vi "Circular.vi"(5 "Direction":u16(ring) items=["Clockwise", "Counter-clockwise"], 7 "Speed":dbl, 8 "error in (no error)":errorcluster, 9 "XY End":dbl[](array[numeric]), 10 "XY Center":dbl[](array[numeric]), 11 "Gantry in":refnum<class "A3200.lvclass">) -> (0 "error out":errorcluster, 3 "Gantry out":refnum<class "A3200.lvclass">)   [LabVIEW 2016, in "A3200.lvclass"]
uses:
  A3200.lvclass
  A3200.lvclass/A3200.ctl
  <userlib>/Aerotech A3200.lnk/Aerotech VIs.lvlib
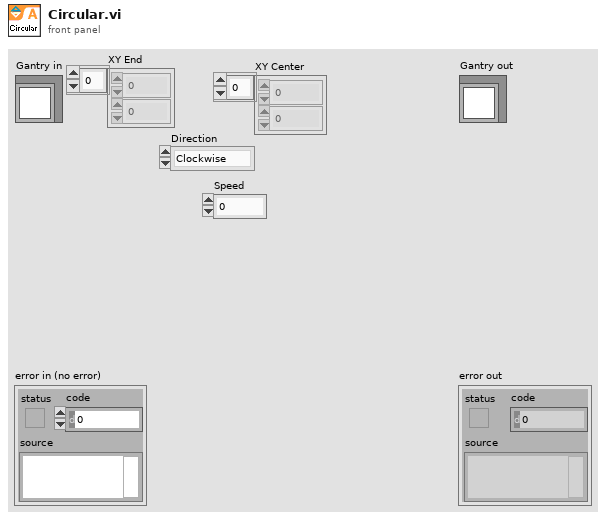
[diagram p1: front panel]
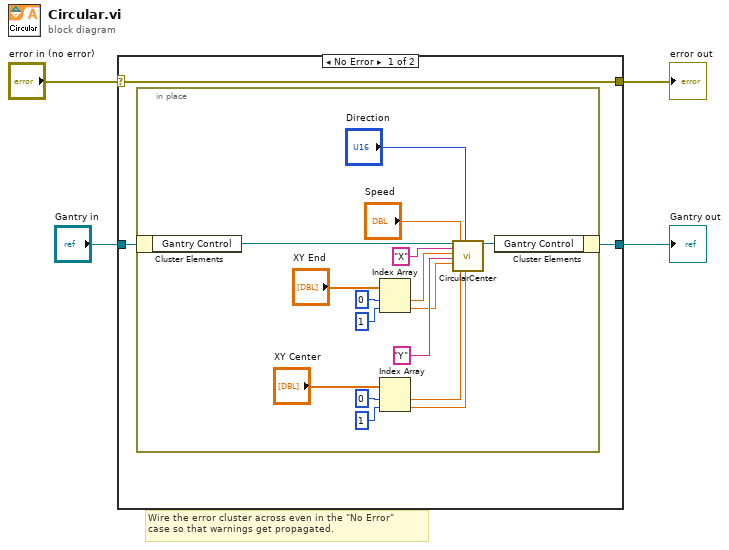
[diagram p0: block diagram]
diagram:
  # "Wire the error cluster across even in the \"No Error\"\ncase so that warnings get propagated."
  n1 = case shown="No Error" "error in (no error)" {
    selector: "error in (no error)" -> [w7 w25]
    tunnel: [w7 w25] -> w3
    tunnel: [w5 w24] -> w1
    tunnel: "Gantry in" -> [w6 w24]
    frame No Error {
      n2 = in-place {
        n3 = in-place-cluster #1(w6) -> ("Gantry Control"=w15:refnum<k24>)
        n4 = Index Array(array="XY End", index #1=0 ("index"), index #2=1 ("index")) -> (element #1=w17:dbl, element #2=w16:dbl)
        n5 = Index Array(array="XY Center", index #1=0 ("index"), index #2=1 ("index")) -> (element #1=w21:dbl, element #2=w20:dbl)
        n6 = call <userlib>:"CircularCenter.vi"("controller in"=w15, "axis 1 name"="X", "axis 1 endpoint"=w17, "axis 2 name"="Y" ("axis 1 name"), "axis 2 endpoint"=w16, "speed"="Speed", "axis 1 center point"=w21, "direction"="Direction", "axis 2 center point"=w20) -> ("controller out"=w14:refnum<k24>)  [unwired: 9 in, 1 out]
        n7 = in-place-cluster #1("Gantry Control"=w14) -> (w5:refnum<class "A3200.lvclass">)
      }
    }
    frame Error {
    }
  }
  "error out" <- w3
  "Gantry out" <- w1
